vi "cm2nm_add_session_to_sample_table.vi"(2 "Sample locations of Interest":refnum<vi>, 3 "Session Name/ID_out":string) -> ()   [LabVIEW 2011]
doc: "Add the session to the row of sessions in the session table sent as a reference."
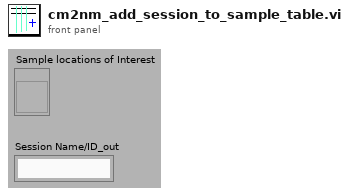
[diagram p1: front panel]
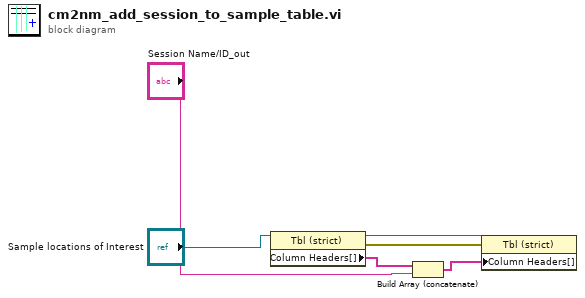
[diagram p0: block diagram]
diagram:
  n1 = property on="Property Node" class="Tbl (strict)"(reference="Sample locations of Interest") -> (reference out=w1:refnum<vi>, error out=w2:errorcluster, "Column Headers[]"=w4:string[])  [unwired: 1 in]
  n2 = Build Array (concatenate)(w4, "Session Name/ID_out") -> (w3:string[])
  n3 = property on="Property Node" class="Tbl (strict)"(reference=w1, error in=w2, "Column Headers[]"=w3) -> ()  [unwired: 2 out]
